vi "Modbus RT Driver VI Modbus - Get Status.vi"(7 "DEBUG General Settings":T2={"Communication_Type"=0, "Modbus_Type"=0, "Read_Write_Loop_Period"=-1, "TCP Settings"={"TCP_Settings_Port"=0, "TCP_Settings_IP_Timeout"=0, "TCP_Settings_IP_Slave_Address"=""}, "Serial Settings"={"Serial_Settings_Flow_Control"=0, "Serial_Settings_Baud_Rate"=0, "Serial_Settings_Parity"=0, "Serial_Settings_Resource_Name"="", "Serial_Settings_Serial_Type"=0, "Serial_Settings_Unit_ID"=0}} {"Communication_Type" items=["TCP", "Serial"]; "Modbus_Type" items=["Master", "Slave"]; "Serial Settings"."Serial_Settings_Flow_Control" items=["None", "XONXOFF", "RTSCTS", "XONXOFFANDRTSCTS", "DTRDSR", "XONXOFFANDDTRDSR"]; "Serial Settings"."Serial_Settings_Parity" items=["None", "Odd", "Even"]; "Serial Settings"."Serial_Settings_Serial_Type" items=["RTU", "ASCII"]}, 8 "error in (no error)":errorcluster, 9 "State In":T1, 11 "ModbusPharLap.lvlibp:Modbus API":refnum<class "Modbus API.lvclass">) -> (0 "error out":errorcluster, 1 "?":T1, 2 "Array":dbl[](array[numeric]), 3 "ModbusPharLap.lvlibp:Modbus API":refnum<class "Modbus API.lvclass">)   [LabVIEW 2014, in "Modbus Engine.lvlib"]
uses:
  Modbus Engine.lvlib
  ModbusPharLap.lvlibp/Modbus Library/API/Modbus API.lvclass
  XML Deserializer/XML VIs/API/Controls/Modbus_General_Settings.ctl
  XML Deserializer/XML VIs/API/Controls/Modbus_Communication_Type.ctl
  XML Deserializer/XML VIs/API/Controls/Modbus_Type.ctl
  XML Deserializer/XML VIs/API/Controls/Modbus_Serial_Settings_Flow_Control.ctl
  XML Deserializer/XML VIs/API/Controls/Modbus_Serial_Settings_Parity.ctl
  XML Deserializer/XML VIs/API/Controls/Modbus_Serial_Settings_Serial_Type.ctl
  Modbus RT Driver VI States Definition.ctl
  ModbusPharLap.lvlibp/Modbus Library/API/Slave/Modbus Slave.lvclass
  Shared/Modbus Shared.lvlib
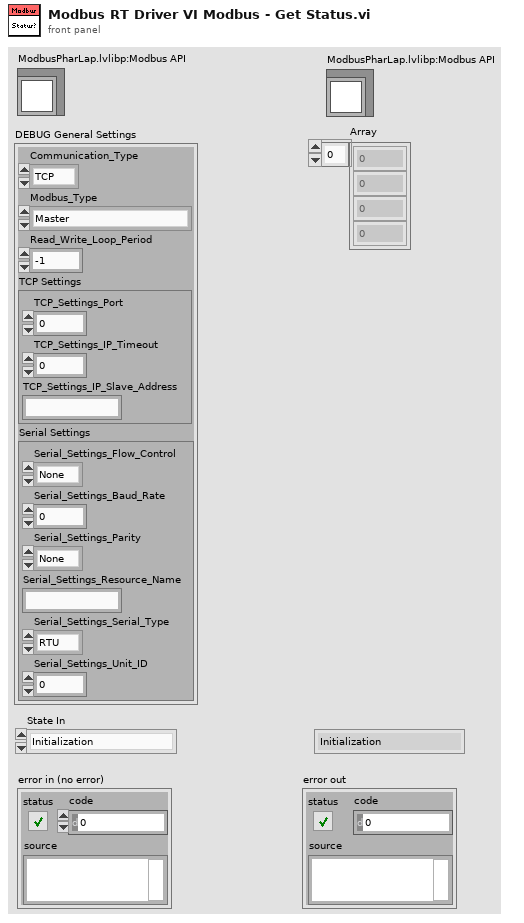
[diagram p1: front panel]
types:
  T1 = typedef "Modbus Engine.lvlib/Modbus RT Driver VI States Definition.ctl" = enum16{"Initialization", "Master - Connect", "Slave - Create Instance", "Exit", "Connected"}
  T2 = typedef "Modbus Shared.lvlib/Modbus_General_Settings.ctl" = cluster{"Communication_Type":T3, "Modbus_Type":T4, "Read_Write_Loop_Period":i64, "TCP Settings":cluster{"TCP_Settings_Port":u16, "TCP_Settings_IP_Timeout":u32, "TCP_Settings_IP_Slave_Address":string}, "Serial Settings":cluster{"Serial_Settings_Flow_Control":T5, "Serial_Settings_Baud_Rate":u32, "Serial_Settings_Parity":T6, "Serial_Settings_Resource_Name":string, "Serial_Settings_Serial_Type":T7, "Serial_Settings_Unit_ID":u8}}
  T3 = typedef "Modbus Shared.lvlib/Modbus_Communication_Type.ctl" = i32
  T4 = typedef "Modbus Shared.lvlib/Modbus_Type.ctl" = i32
  T5 = typedef "Modbus Shared.lvlib/Modbus_Serial_Settings_Flow_Control.ctl" = i32
  T6 = typedef "Modbus Shared.lvlib/Modbus_Serial_Settings_Parity.ctl" = i32
  T7 = typedef "Modbus Shared.lvlib/Modbus_Serial_Settings_Serial_Type.ctl" = i32
  T8 = typedef "ModbusPharLap.lvlibp/Network Slave.lvclass/daemon status.ctl" = enum16{"Not Started", "Running", "Error", "Stopped"}
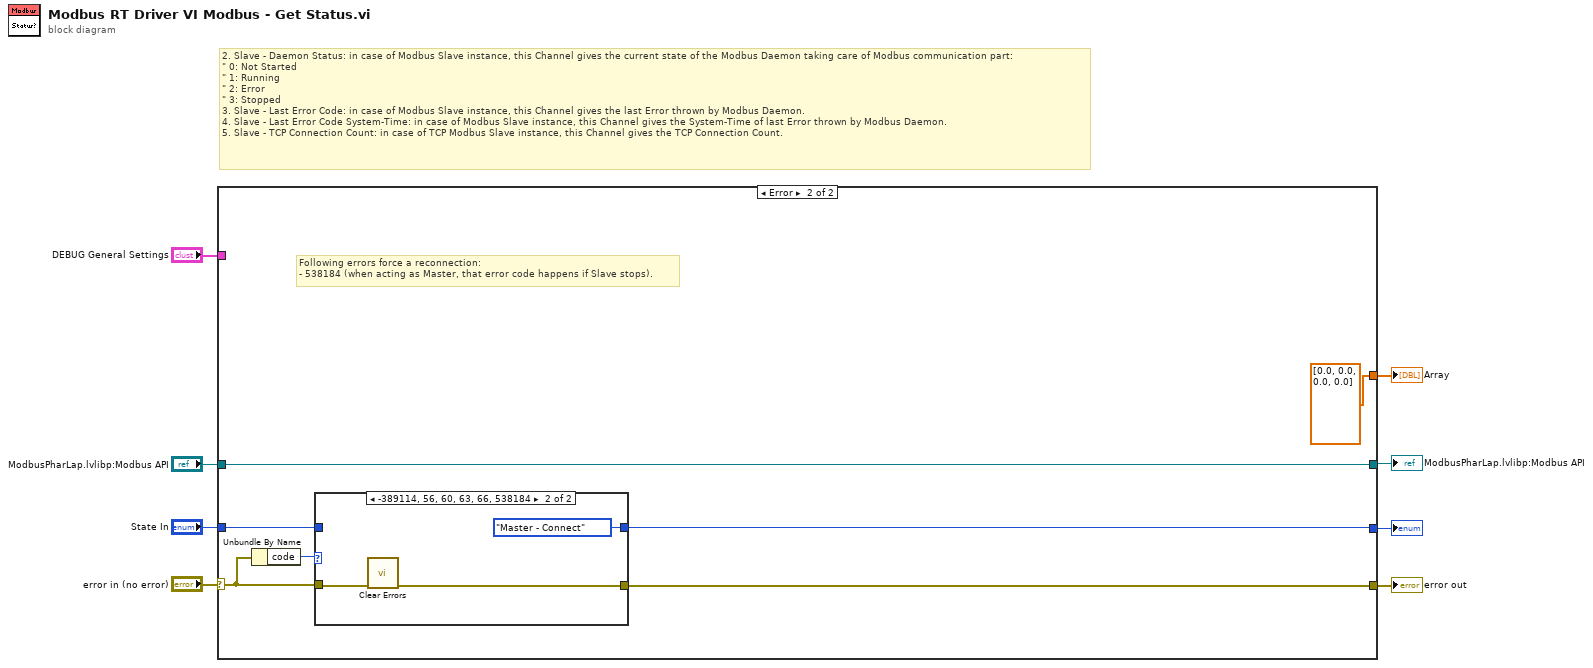
[diagram p0: block diagram]
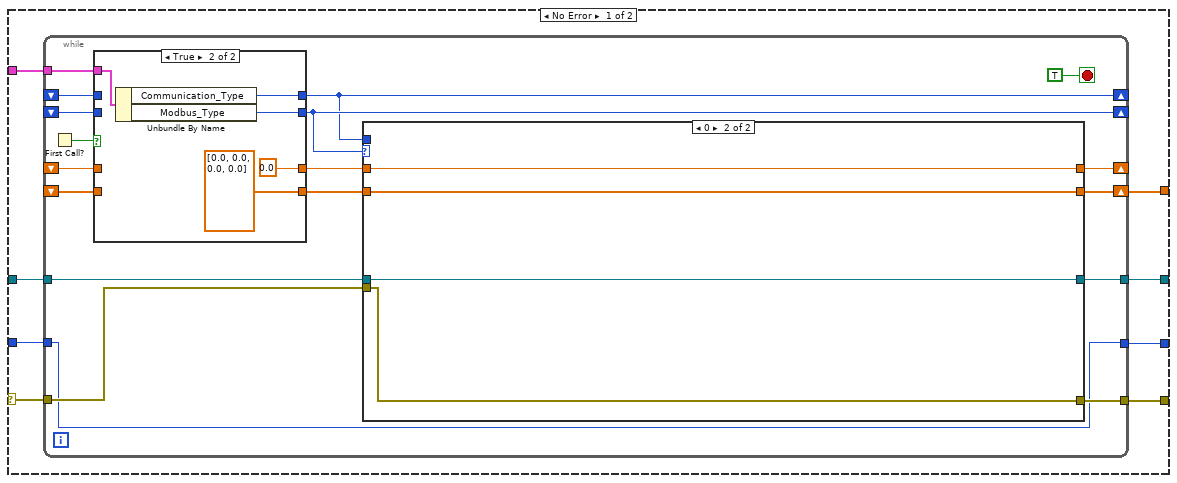
[diagram p2: hidden frame]
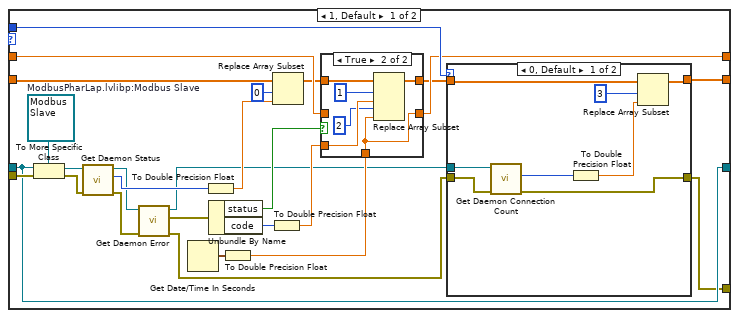
[diagram p3: hidden frame]
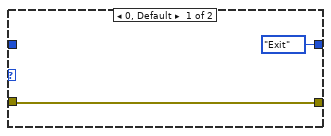
[diagram p7: hidden frame]
diagram:
  # "2. Slave - Daemon Status: in case of Modbus Slave instance, this Channel gives the current state of the Modbus Daemon taking care of Modbus communication part:\n\"\t0: Not Started\n\"\t1: Running\n\"\t2: Error\n\"\t3: Stopped\n3. Slave - Last Error Code: in case of Modbus Slave instance, this Channel gives the last Error thrown by Modbus Daemon.\n4. Slave - Last Error Code System-Time: in case of Modbus Slave instance, this Channel gives the System-Time of last Error thrown by Modbus Daemon.\n5. Slave - TCP Connection Count: in case of TCP Modbus Slave instance, this Channel gives the TCP Connection Count."
  n1 = case shown="Error" "error in (no error)" {
    selector: "error in (no error)" -> [w14 w96]
    tunnel: [w16 w95] -> w8
    tunnel: [w12 w98] -> w4
    tunnel: "ModbusPharLap.lvlibp:Modbus API" -> [w15 w98]
    tunnel: "DEBUG General Settings" -> [w13 _]
    tunnel: "State In" -> [w11 w94]
    tunnel: [w10 w93] -> w2
    tunnel: [w9 dbl[] [0.0, 0.0, 0.0, 0.0]] -> w1
    frame No Error {
      n2 = while {
        tunnel: [w34] -> w16
        tunnel: w15 -> [w33]
        tunnel: w14 -> [w32]
        shift-right: [w19] -> w9
        shift-left: _ -> [w30]
        shift-right: [w21] -> _
        shift-left: _ -> [w29]
        tunnel: w13 -> [w28]
        shift-right: [w23] -> _
        shift-left: _ -> [w27]
        shift-right: [w24] -> _
        shift-left: _ -> [w26]
        tunnel: [w18] -> w12
        tunnel: w11 -> [w17]
        tunnel: [w17] -> w10
        stop <- TRUE stop-if-true
        n3 = First Call?() -> (First Call?: T/F=w31:bool)
        n4 = case shown="True" w31 {
          tunnel: [w86 dbl[] [0.0, 0.0, 0.0, 0.0]] -> w20
          tunnel: w30 -> [w86 _]
          tunnel: w29 -> [w83 _]
          tunnel: [w83 0.0] -> w22
          tunnel: w28 -> [_ w89]
          tunnel: [w85 w88] -> w23
          tunnel: [w84 w87] -> w24
          tunnel: w27 -> [w85 _]
          tunnel: w26 -> [w84 _]
          frame False {
          }
          frame True {
            n5 = Unbundle By Name(w89) -> ("Communication_Type"=w88:T3, "Modbus_Type"=w87:T4)
          }
        }
        n6 = case shown="0" w24 {
          tunnel: [w52 w79] -> w34
          tunnel: w33 -> [w53 w80]
          tunnel: w32 -> [w59 w79]
          tunnel: w23 -> [w55 _]
          tunnel: w22 -> [w50 w82]
          tunnel: [w49 w82] -> w21
          tunnel: w20 -> [w58 w81]
          tunnel: [w54 w81] -> w19
          tunnel: [w53 w80] -> w18
          frame 1, Default {
            w35 = refnum<class "Modbus Slave.lvclass"> refnum  # ModbusPharLap.lvlibp:Modbus Slave
            n7 = To More Specific Class(target class=w35, reference=w53, error in=w59) -> (specific class reference=w43:refnum<class "Modbus Slave.lvclass">, error out=w42:errorcluster)
            n8 = call-dynamic "Get Daemon Status.vi"("error in (no error)"=w42, "Modbus slave in"=w43) -> ("error out"=w38:errorcluster, "daemon status"=w41:T8, "Modbus Slave out"=w40:refnum<class "Modbus Slave.lvclass">)  [unwired: 7 in]
            n9 = call-dynamic "Get Daemon Error.vi"("error in (no error)"=w38, "Modbus slave in"=w40) -> ("error out"=w37:errorcluster, "daemon error"=w39:errorcluster, "Modbus Slave out"=w36:refnum<class "Modbus Slave.lvclass">)  [unwired: 7 in]
            n10 = Get Date/Time In Seconds() -> (seconds since 1Jan1904=w60:timestamp)
            n11 = To Double Precision Float(number=w41) -> (double precision float=w56:dbl)
            n12 = Unbundle By Name(w39) -> ("status"=w44:bool, "code"=w51:i32)
            n13 = To Double Precision Float(number=w60) -> (double precision float=w46:dbl)
            n14 = To Double Precision Float(number=w51) -> (double precision float=w45:dbl)
            n15 = Replace Array Subset(array=w58, new element=w56, index=0) -> (w48:dbl[])
            n16 = case shown="True" w44 {
              tunnel: w50 -> [w61 _]
              tunnel: [w61 w63] -> w49
              tunnel: w48 -> [w62 w67]
              tunnel: [w62 w68] -> w47
              tunnel: w46 -> [_ w63]
              tunnel: w45 -> [_ w65]
              frame False {
              }
              frame True {
                n17 = Replace Array Subset(array=w67, new element #1=w65, index #1=1 ("index"), new element #2=w63, index #2=2 ("index")) -> (w68:dbl[])
              }
            }
            n18 = case shown="0, Default" w55 {
              tunnel: w47 -> [w76 w78]
              tunnel: [w75 w78] -> w54
              tunnel: w36 -> [w72 _]
              tunnel: w37 -> [w71 w77]
              tunnel: [w69 w77] -> w52
              frame 0, Default {
                n19 = call-dynamic "Get Daemon Connection Count.vi"("error in (no error)"=w71, "Modbus slave in"=w72) -> ("error out"=w69:errorcluster, "connection count"=w70:u32)  [unwired: 7 in, 1 out]
                n20 = To Double Precision Float(number=w70) -> (double precision float=w73:dbl)
                n21 = Replace Array Subset(array=w76, new element=w73, index=3) -> (w75:dbl[])
              }
              frame 1 {
              }
            }
          }
          frame 0 {
          }
        }
      }
    }
    frame Error {
      # "Following errors force a reconnection:\n- 538184 (when acting as Master, that error code happens if Slave stops)."
      n22 = Unbundle By Name(w96) -> ("code"=w97:i32)
      n23 = case shown="-389114, 56, 60, 63, 66, 538184" w97 {
        tunnel: w96 -> [w100 w103]
        tunnel: [w100 w102] -> w95
        tunnel: w94 -> [_ _]
        tunnel: [Modbus_RT_Driver_VI_States_Definition."Exit" ("State In") Modbus_RT_Driver_VI_States_Definition."Master - Connect" ("State In")] -> w93
        frame 0, Default {
        }
        frame -389114, 56, 60, 63, 66, 538184 {
          n24 = call <vilib>:"Clear Errors.vi"("error in (no error)"=w103) -> ("error out"=w102:errorcluster)  [unwired: 5 in, 1 out]
        }
      }
    }
  }
  "error out" <- w8
  "Array" <- w1
  "ModbusPharLap.lvlibp:Modbus API" <- w4
  "?" <- w2
